vi "TDC_数据修正.vi"(1 "细计数输入":dbl[](array[numeric])) -> (0 "修正后的细计数":dbl[](array[numeric]))   [LabVIEW 2014]
panel:
  out "积分表":dbl[](graph)
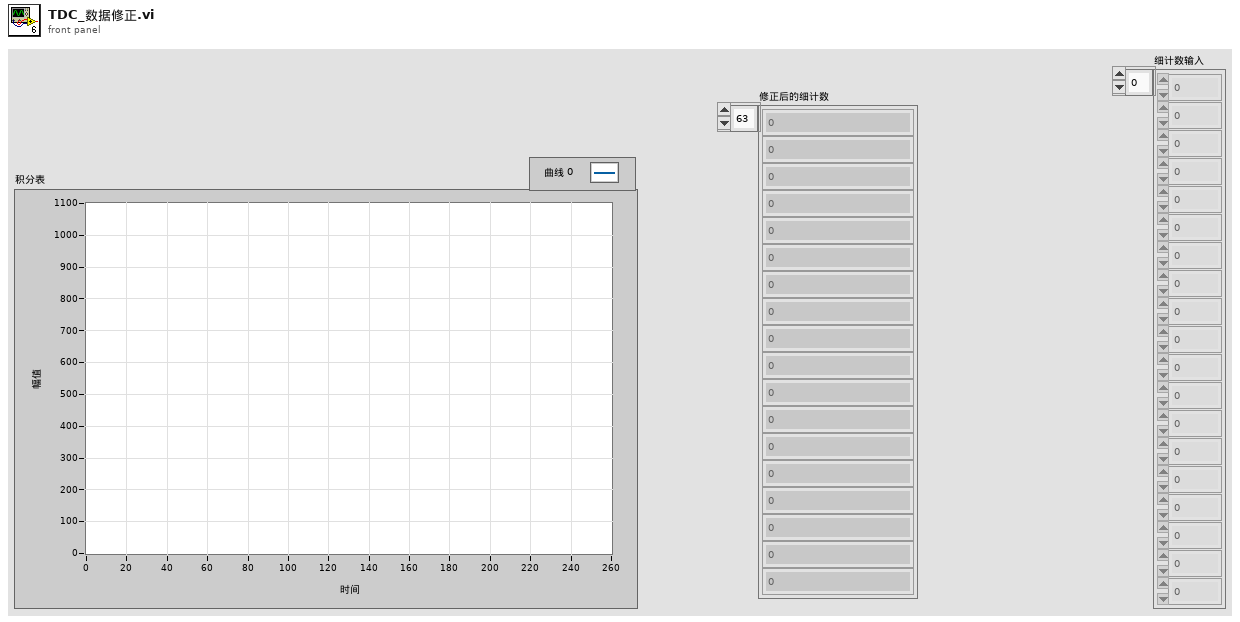
[diagram p1: front panel]
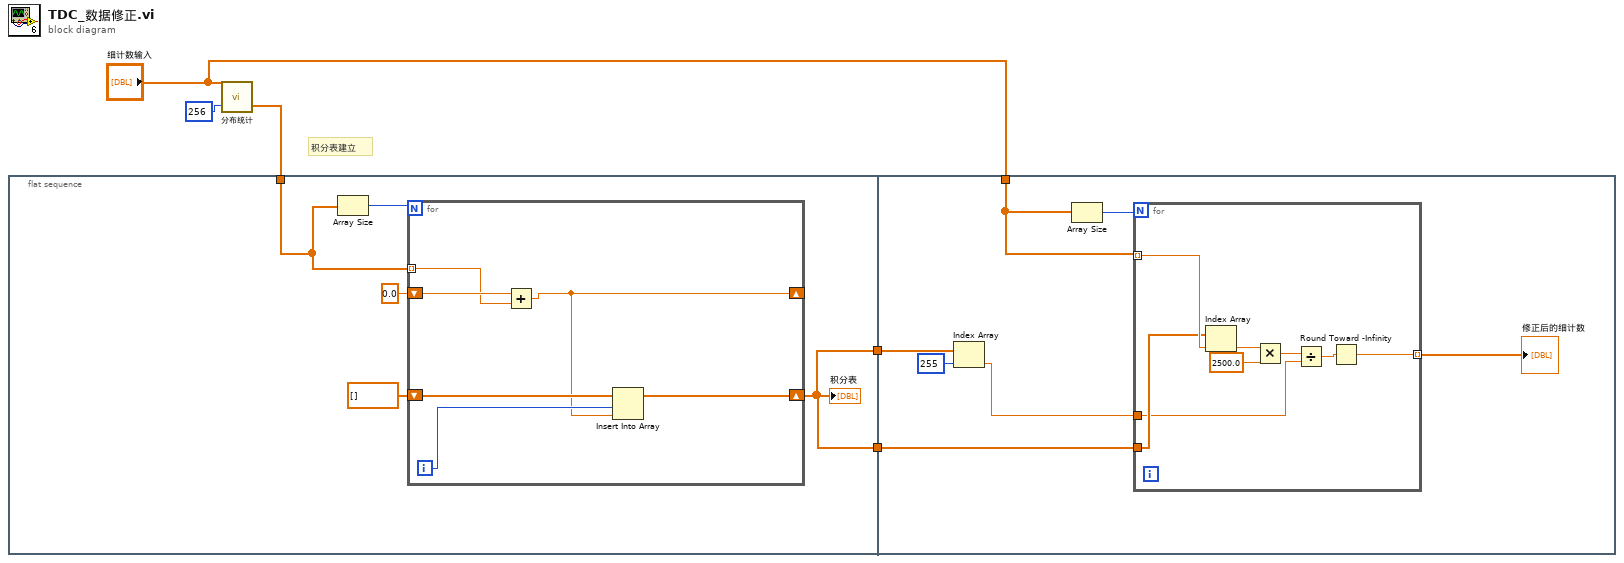
[diagram p0: block diagram]
diagram:
  # "积分表建立"
  n1 = flat-sequence {
    tunnel: [w6] -> w5
    tunnel: w3 -> [w7]
    tunnel: [w6] -> w2
    tunnel: w5 -> [w22]
    tunnel: "细计数输入" -> [w21]
    tunnel: w2 -> [w20]
    frame #0 {
      n2 = Array Size(array=w7) -> (size(s)=w10:i32)
      n3 = for {
        N: w10 -> [_]
        shift-right: [w11] -> _
        shift-left: 0.0 -> [w16]
        tunnel: w7 -> [w15] mode=indexing
        shift-right: [w13] -> w6
        shift-left: dbl[] [] -> [w14]
        i -> [w12]
        n4 = Add(x=w16, y=w15) -> (x+y=w11:dbl)
        n5 = Insert Into Array(array=w14, index=w12, new element=w11) -> (w13:dbl[])
      }
      "积分表" <- w6
    }
    frame #1 {
      n6 = Index Array(array=w20, index=255 ("索引")) -> (element=w18:dbl)
      n7 = Array Size(array=w21) -> (size(s)=w23:i32)
      n8 = for {
        N: w23 -> [_]
        tunnel: w22 -> [w30]
        tunnel: w21 -> [w31] mode=indexing
        tunnel: w18 -> [w26]
        tunnel: [w24] -> w17 mode=indexing
        n9 = Index Array(array=w30, index=w31) -> (element=w29:dbl)
        n10 = Multiply(x=w29, y=2500.0) -> (x*y=w27:dbl)
        n11 = Divide(x=w27, y=w26) -> (x/y=w25:dbl)
        n12 = Round Toward -Infinity(1:w25) -> (0:w24:dbl)
      }
      "修正后的细计数" <- w17
    }
  }
  n13 = call "分布统计.vi"("道数"=256, "数组"="细计数输入") -> ("分布谱"=w3:dbl[])  [unwired: 1 out]
